vi "Victor8246_Config.vi"(0 "参数":T1, 11 "错误输入":errorcluster caption="错误输入（无错误）") -> (4 "VISA资源":refnum<visa-resource-name>, 10 "OK?":bool, 15 "错误输出":errorcluster)   [LabVIEW 2015, in "Victor8246.lvlib"]
uses:
  Victor8246.lvlib
  <vilib>/Instr/_visa.llb/VISA Configure Serial Port (Instr).vi
panel:
  in  "MyIndex":u8
  # "频率，电容没有高速 。"
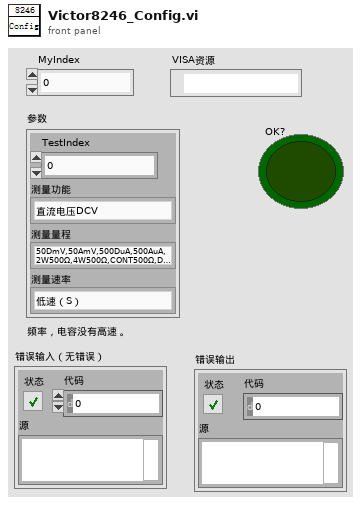
[diagram p1: front panel]
types:
  T1 = cluster{"TestIndex":i32, "测量功能":enum16{"直流电压DCV", "交流电压ACV", "直流电流DCI", "交流电流ACI", "电阻OHM_2W", "电阻OHM_4W", "通断测试CONT", "二极管DIODE", "频率FREQ", "电容CAP", "温度TEMP", "热电阻RTD", "分贝dBm"}, "测量量程":enum16{"50DmV,50AmV,500DuA,500AuA,2W500Ω,4W500Ω,CONT500Ω,DIODE2V,10Hz,10nF,K,PT100,db", "500DmV,500AmV,5000DuA,5000AuA,2W5kΩ,4W5kΩ,100Hz,100nF", "5DV,5AV,50DmA,50AmA,2W50kΩ,4W50kΩ,1000Hz,1000nF", "50DV,50AV,500DmA,500AmA,2W500kΩ,4W500kΩ,10kHz,10μF", "500DV,500AV,5DA,5AA,2W5MΩ,4W5MΩ,100kHz,100μF", "1000DV，1000AV,10DA,10AA,2W50MΩ,4W50MΩ,1000kHz,1000μF", "10MHz，100mF", "占空比DUTY，100mF"}, "测量速率":enum16{"低速（S）", "高速（F）"}}
  T2 = enum16{"直流电压DCV", "交流电压ACV", "直流电流DCI", "交流电流ACI", "电阻OHM_2W", "电阻OHM_4W", "通断测试CONT", "二极管DIODE", "频率FREQ", "电容CAP", "温度TEMP", "热电阻RTD", "分贝dBm"}
  T3 = enum16{"50DmV,50AmV,500DuA,500AuA,2W500Ω,4W500Ω,CONT500Ω,DIODE2V,10Hz,10nF,K,PT100,db", "500DmV,500AmV,5000DuA,5000AuA,2W5kΩ,4W5kΩ,100Hz,100nF", "5DV,5AV,50DmA,50AmA,2W50kΩ,4W50kΩ,1000Hz,1000nF", "50DV,50AV,500DmA,500AmA,2W500kΩ,4W500kΩ,10kHz,10μF", "500DV,500AV,5DA,5AA,2W5MΩ,4W5MΩ,100kHz,100μF", "1000DV，1000AV,10DA,10AA,2W50MΩ,4W50MΩ,1000kHz,1000μF", "10MHz，100mF", "占空比DUTY，100mF"}
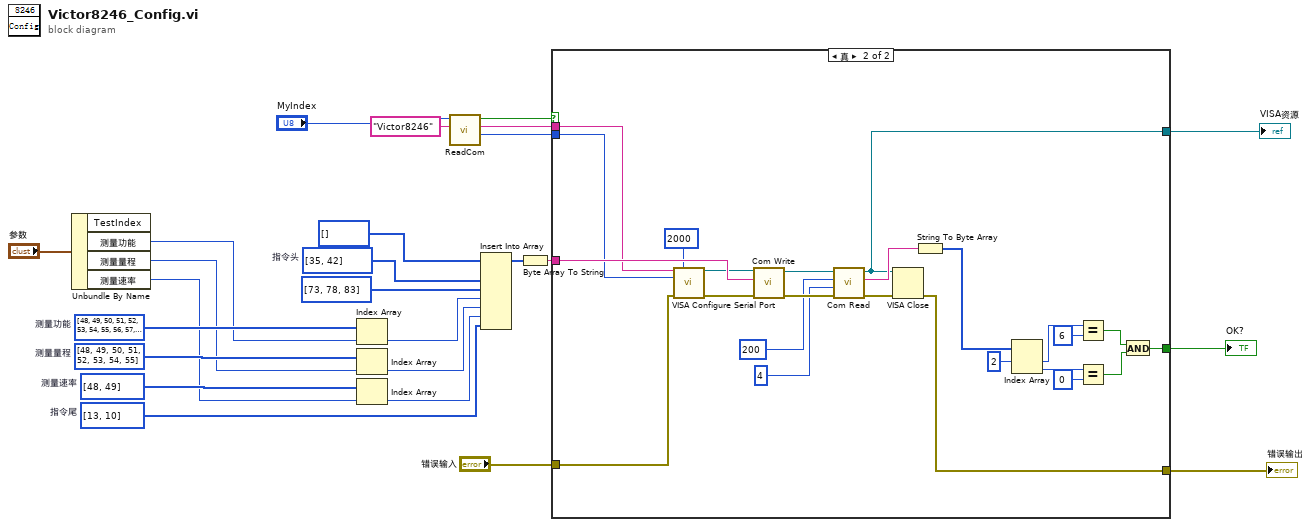
[diagram p0: block diagram]
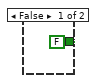
[diagram p2: hidden frame]
diagram:
  w15 = u8[] [48, 49]  # 测量速率
  w17 = u8[] [48, 49, 50, 51, 52, 53, 54, 55]  # 测量量程
  w19 = u8[] [48, 49, 50, 51, 52, 53, 54, 55, 56, 57, 58, 171, 60]  # 测量功能
  w20 = u8[] [13, 10]  # 指令尾
  w25 = u8[] [35, 42]  # 指令头
  n1 = Unbundle By Name("参数") -> ("测量功能"=w10:T2, "测量量程"=w9:T3, "测量速率"=w8:enum16{"低速（S）", "高速（F）"})  [unwired: 1 out]
  n2 = Index Array(array=w19, index=w10) -> (element=w18:u8)
  n3 = Index Array(array=w17, index=w9) -> (element=w16:u8)
  n4 = Index Array(array=w15, index=w8) -> (element=w14:u8)
  n5 = call "ReadCom.vi"("仪器名称"="Victor8246", "MyIndex"="MyIndex") -> ("Baudrate"=w4:i32, "COM"=w5:string, "OK?"=w3:bool)  [unwired: 7 in]
  n6 = Insert Into Array(array=u8[] [] ("数组"), new element #1=w25, new element #2=u8[] [73, 78, 83], new element #3=w18, new element #4=w16, new element #5=w14, new element #6=w20) -> (w23:u8[])  [unwired: 1 in]
  n7 = Byte Array To String(unsigned byte array=w23) -> (string=w12:string)
  n8 = case shown="真" w3 {
    tunnel: [FALSE w43] -> w22
    tunnel: "错误输入" -> [_ w41]
    tunnel: w12 -> [_ w40]
    tunnel: w5 -> [_ w32]
    tunnel: w4 -> [_ w31]
    tunnel: [_ w28] -> w2
    tunnel: [_ w27] -> w1
    frame False {
    }
    frame True {
      n9 = call-poly "VISA Configure Serial Port"("VISA resource name"=w32, "timeout (10sec)"=u32 2000, "baud rate (9600)"=w31, "error in (no error)"=w41) -> ("VISA resource name out"=w29:refnum<visa-resource-name>, "error out"=w33:errorcluster)  [unwired: 10 in]
      n10 = call "Com Write.vi"("错误输入（无错误）"=w33, "Wbuff"=w40, "VISA In"=w29) -> ("错误输出"=w39:errorcluster, "VISA Out"=w38:refnum<visa-resource-name>)  [unwired: 7 in]
      n11 = call "Com Read.vi"("错误输入（无错误）"=w39, "num"=u32 4, "超时"=u32 200, "VISA In"=w38) -> ("错误输出"=w34:errorcluster, "buff"=w35:string, "VISA Out"=w27:refnum<visa-resource-name>)  [unwired: 5 in]
      n12 = VISA Close(VISA resource name=w27, error in (no error)=w34) -> (error out=w28:errorcluster)
      n13 = String To Byte Array(string=w35) -> (unsigned byte array=w42:u8[])
      n14 = Index Array(array=w42, index #1=2 ("索引")) -> (element #1=w49:u8, element #2=w46:u8)  [unwired: 1 in]
      n15 = Equal?(x=w49, y=u8 6) -> (x = y?=w45:bool)
      n16 = Equal?(x=w46, y=u8 0) -> (x = y?=w44:bool)
      n17 = And(x=w45, y=w44) -> (x .and. y?=w43:bool)
    }
  }
  "OK?" <- w22
  "错误输出" <- w2
  "VISA资源" <- w1
